vi "init.vi"(10 "Rx UDP Config":T1={"Local UDP Port (Tx)"=1002, "Remote IP (Rx)"="localhost", "Remote UDP Port (Rx)"=1234, "Timeout [ms]"=1}) -> (0 "error out":errorcluster, 3 "UDP Out":refnum<class "UDP Rx.lvclass">)   [LabVIEW 2012, in "UDP Rx.lvclass"]
uses:
  UDP Rx.lvclass
  UDP Rx.lvclass/UDP Rx.ctl
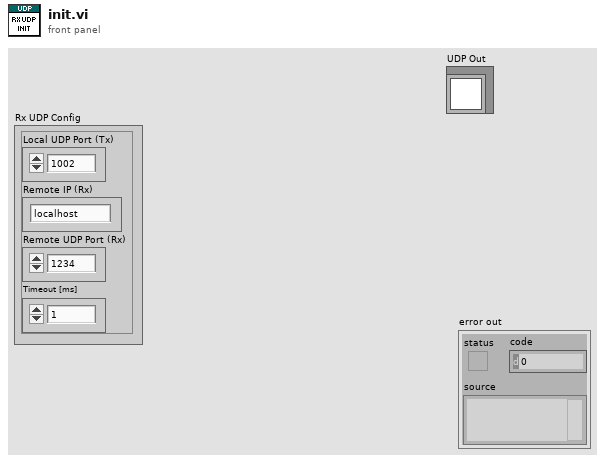
[diagram p1: front panel]
types:
  T1 = cluster{"Local UDP Port (Tx)":u16, "Remote IP (Rx)":string, "Remote UDP Port (Rx)":u16, "Timeout [ms]":u16}
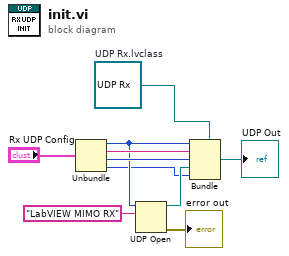
[diagram p0: block diagram]
diagram:
  w2 = refnum<class "UDP Rx.lvclass"> refnum  # UDP Rx.lvclass
  n1 = Unbundle "Unbundle"("Rx UDP Config") -> ("Local UDP Port (Tx)"=w4:u16, "Remote IP (Rx)"=w9:string, "Remote UDP Port (Rx)"=w8:u16, "Timeout [ms]"=w3:u16)
  n2 = UDP Open(10:"LabVIEW MIMO RX" ("service name"), 11:w4) -> (port=w7:refnum<k16>, 0:→"error out":errorcluster)  [unwired: 3 in, 1 out]
  n3 = Bundle(cluster=w2, w4, w9, w8, w7, w3) -> (→"UDP Out":refnum<class "UDP Rx.lvclass">)
